vi "finalizeScript.vi"(8 "error in (no error)":errorcluster, 11 "K2602 in":refnum<class "K2602.lvclass">) -> (0 "error out":errorcluster, 2 "script":string, 3 "K2602 out":refnum<class "K2602.lvclass">)   [LabVIEW 2011, in "Hardware.lvlib" / "Channels.lvlib" / "K2602.lvclass"]
uses:
  K2602.lvclass
  K2602.lvclass/K2602.ctl
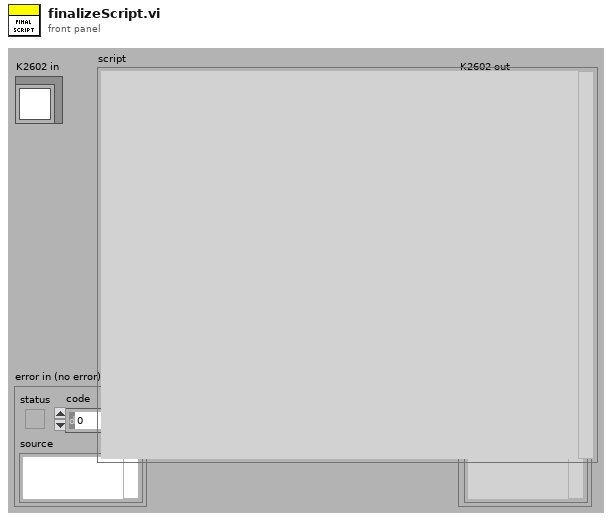
[diagram p1: front panel]
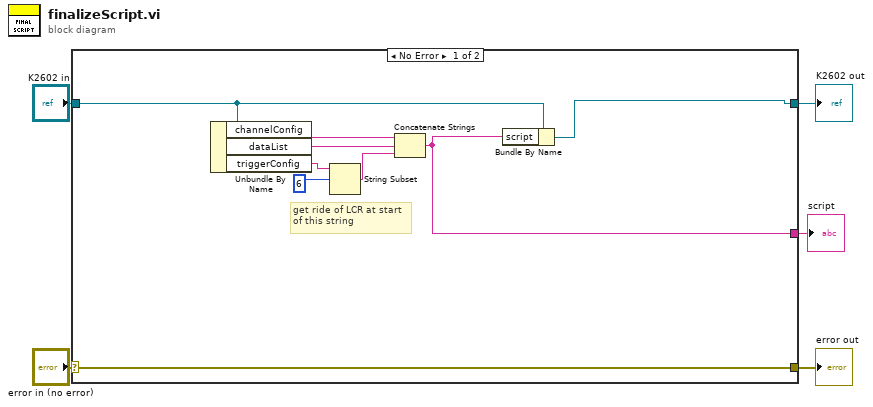
[diagram p0: block diagram]
diagram:
  n1 = case shown="No Error" "error in (no error)" {
    selector: "error in (no error)" -> [w14 w16]
    tunnel: [w14 w16] -> w4
    tunnel: [w12 w15] -> w2
    tunnel: "K2602 in" -> [w13 w15]
    tunnel: [w6 _] -> w1
    frame No Error {
      # "get ride of LCR at start\nof this string"
      n2 = Unbundle By Name(w13) -> ("channelConfig"=w9:string, "dataList"=w8:string, "triggerConfig"=w11:string)
      n3 = String Subset(string=w11, offset (0)=6) -> (substring=w7:string)  [unwired: 1 in]
      n4 = Concatenate Strings(w9, w8, w7) -> (w6:string)
      n5 = Bundle By Name(cluster=w13, "script"=w6) -> (w12:refnum<class "K2602.lvclass">)
    }
    frame Error {
    }
  }
  "error out" <- w4
  "K2602 out" <- w2
  "script" <- w1
